vi "CH_LM Config Display Smoothing Size Time.vi"(0 "Meter Index":i32, 2 "Time / s (0:Auto)":i32, 5 "error in (no error)":errorcluster, 7 "Timeout / ms (3000)":i32=3000, 8 "Action (query)":bool, 9 "Lock Timeout / ms (1000)":i32=1000) -> (11 "Lock timed out":bool, 14 "Meter Index":i32, 16 "Time / s":i32, 19 "error out":errorcluster)   [LabVIEW 2012, in "CH_LM.lvlib"]
doc: "Display data smoothing is controlled differently depending on the type of probe attached.\n\nThis command will set/query the display data smoothing window size expressed in seconds.\n\n<B>Attention:</B> This command will apply only when a thermopile or optical probe is attached in Watts mode."
uses:
  CH_LM.lvlib
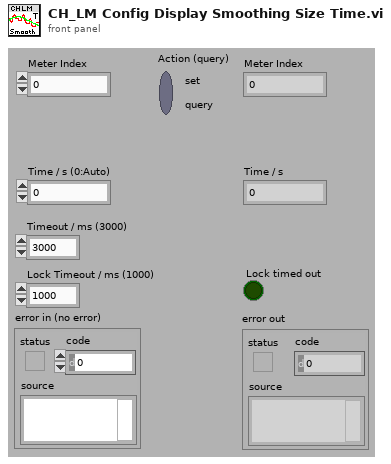
[diagram p1: front panel]
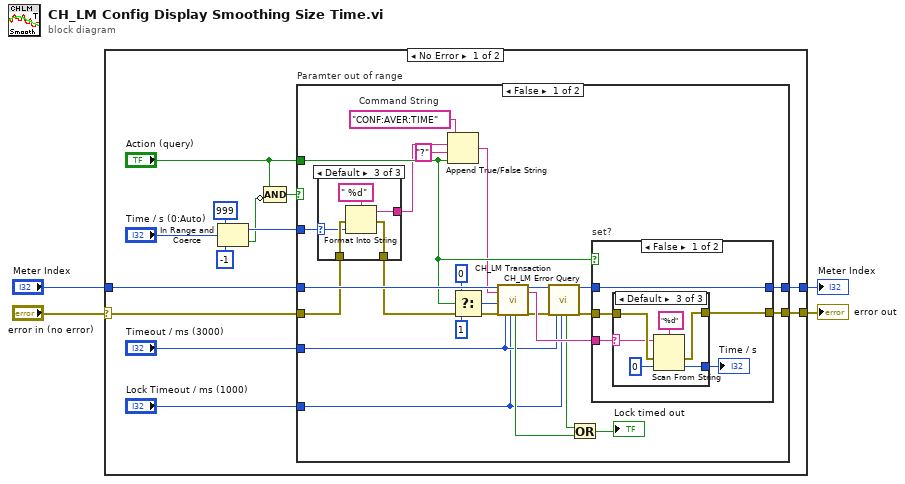
[diagram p0: block diagram]
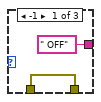
[diagram p2: hidden frame]
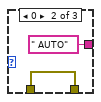
[diagram p3: hidden frame]
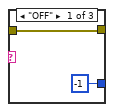
[diagram p4: hidden frame]
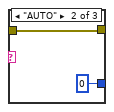
[diagram p5: hidden frame]
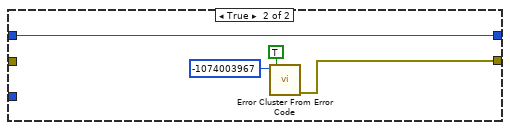
[diagram p7: hidden frame]
diagram:
  n1 = case shown="No Error" "error in (no error)" {
    selector: "error in (no error)" -> [w17 w73]
    tunnel: [w15 w73] -> w4
    tunnel: "Meter Index" -> [w16 w72]
    tunnel: [w14 w72] -> w1
    frame No Error {
      n2 = In Range and Coerce(upper limit=999, x="Time / s (0:Auto)", lower limit=-1) -> (coerced(x)=w11:i32, In Range?=w5:bool)
      n3 = Compound Arithmetic op=AND("Action (query)", invert w5) -> (w7:bool)
      n4 = case "Paramter out of range" shown="False" w7 {
        tunnel: w17 -> [w22 _]
        tunnel: w16 -> [w41 w71]
        tunnel: [w38 w69] -> w15
        tunnel: [w33 w71] -> w14
        tunnel: "Timeout / ms (3000)" -> [w25 _]
        tunnel: "Lock Timeout / ms (1000)" -> [w24 _]
        tunnel: w11 -> [w18 _]
        tunnel: "Action (query)" -> [w23 _]
        frame False {
          w40 = "CONF:AVER:TIME"  # Command String
          n5 = case shown="Default" w18 {
            selector: w18 -> [_ _ w46]
            tunnel: w22 -> [w42 w45 w49]
            tunnel: [w42 w45 w48] -> w21
            tunnel: [" OFF" " AUTO" w47] -> w19
            frame -1 {
            }
            frame 0 {
            }
            frame Default {
              n6 = Format Into String(format string=" %d", error in=w49, w46) -> (resulting string=w47:string, error out=w48:errorcluster)  [unwired: 1 in]
            }
          }
          n7 = Append True/False String(1:w23, 2:"?" ("true string"), 3:w19, 4:w40) -> (0:w20:string)
          n8 = Select(t=0, s=w23, f=1 ("NofStrings (-1:all)")) -> (s? t:f=w35:i32)
          n9 = call "CH_LM Transaction.vi"("Meter Index"=w41, "Command String"=w20, "NofStrings (-1:all)"=w35, "error in (no error)"=w21, "Timeout / ms (3000)"=w25, "Lock Timeout / ms (1000)"=w24) -> ("Lock timed out"=w27:bool, "Meter Index"=w32:i32, "Response"=w39:string, "error out"=w30:errorcluster)  [unwired: 10 out]
          n10 = call "CH_LM Error Query.vi"("Meter Index"=w32, "error in (no error)"=w30, "Timeout / ms (3000)"=w25, "Lock Timeout / ms (1000)"=w24) -> ("Lock timed out"=w28:bool, "Meter Index"=w31:i32, "error out"=w29:errorcluster)  [unwired: 13 out]
          n11 = Or(x=w28, y=w27) -> (x .or. y?=→"Lock timed out":bool)
          n12 = case "set?" shown="False" w23 {
            tunnel: w39 -> [w52 _]
            tunnel: w29 -> [w55 w67]
            tunnel: [w54 w67] -> w38
            tunnel: w31 -> [w53 w66]
            tunnel: [w53 w66] -> w33
            frame False {
              n13 = case shown="Default" w52 {
                selector: w52 -> [_ _ w60]
                tunnel: w55 -> [w56 w59 w65]
                tunnel: [w56 w59 w64] -> w54
                tunnel: [-1 ("default value 1") 0 ("default value 1") w61] -> w51
                frame "OFF" {
                }
                frame "AUTO" {
                }
                frame Default {
                  n14 = Scan From String(format string="%d", input string=w60, error in=w65, default 1=0 ("default value 1")) -> (error out=w64:errorcluster, output 1=w61:i32)  [unwired: 1 in, 2 out]
                }
              }
              "Time / s" <- w51
            }
            frame True {
            }
          }
        }
        frame True {
          n15 = call <vilib>:"Error Cluster From Error Code.vi"("show call chain? (False)"=TRUE, "error code (0)"=-1074003967) -> ("error out"=w69:errorcluster)  [unwired: 1 in, 6 out]
        }
      }
    }
    frame Error {
    }
  }
  "error out" <- w4
  "Meter Index" <- w1
